vi "GenerateAlotOfSignals.vi"() -> (2 "DAQ":T1 {"data" format="%.2f"; "status" format="%08x"})   [LabVIEW 2014]
doc: "Generate some DAQ data (should later be the benchmark) to test the data historian."
uses:
  HISW/controls/typedef_PAQsample.ctl
  <vilib>/ptbypt/NI_PtbyPt.lvlib
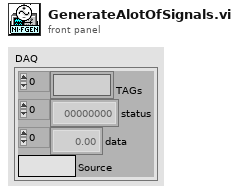
[diagram p1: front panel]
types:
  T1 = typedef "typedef_PAQsample.ctl" = cluster{"TAGs":string[], "status":u32[], "data":dbl[], "Source":string}
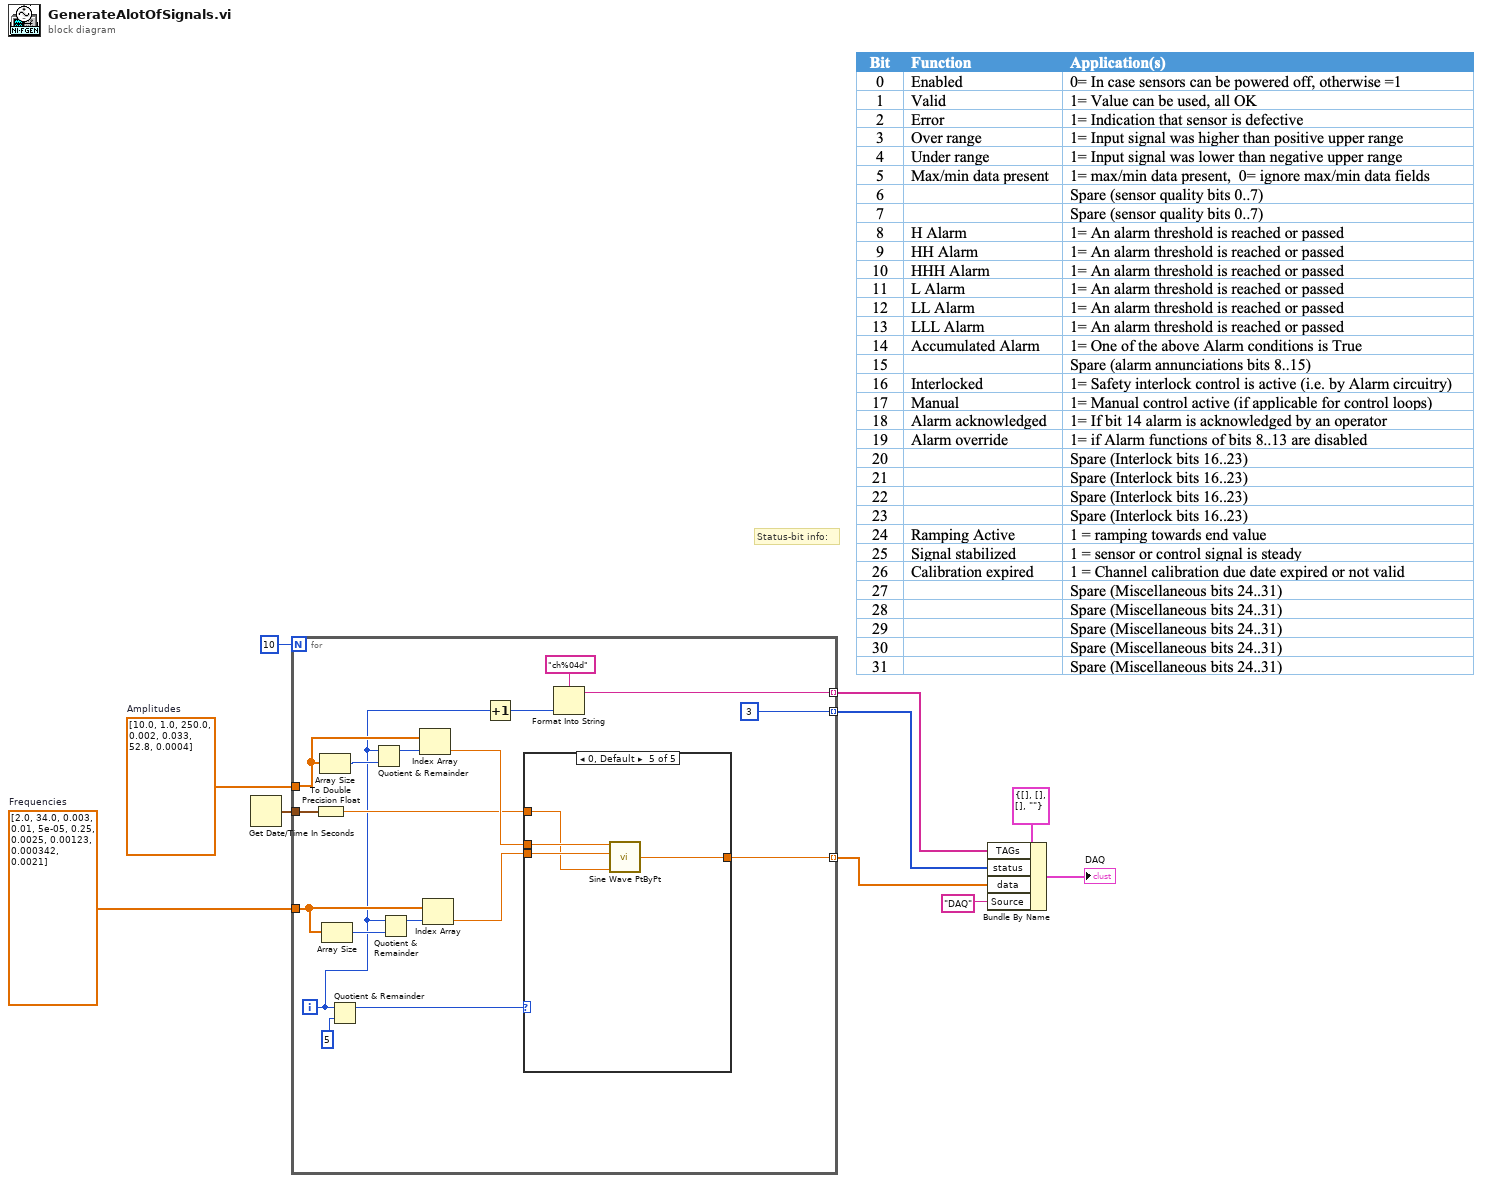
[diagram p0: block diagram]
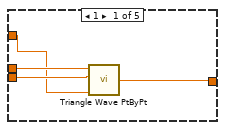
[diagram p2: hidden frame]
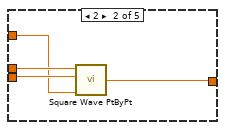
[diagram p3: hidden frame]
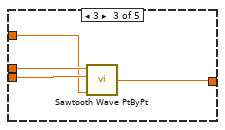
[diagram p4: hidden frame]
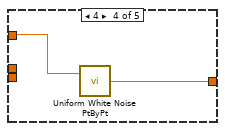
[diagram p5: hidden frame]
diagram:
  w9 = dbl[] [10.0, 1.0, 250.0, 0.002, 0.033, 52.8, 0.0004]  # Amplitudes
  w8 = dbl[] [2.0, 34.0, 0.003, 0.01, 5e-05, 0.25, 0.0025, 0.00123, 0.000342, 0.0021]  # Frequencies
  # "Status-bit info:"
  n1 = Get Date/Time In Seconds() -> (seconds since 1Jan1904=w7:timestamp)
  n2 = for {
    N: 10 -> [_]
    tunnel: w9 -> [w23]
    tunnel: w8 -> [w25]
    tunnel: w7 -> [w18]
    tunnel: [w16] -> w3 mode=indexing
    tunnel: [w12] -> w5 mode=indexing
    tunnel: [u32 3] -> w4 mode=indexing
    i -> [w15]
    n3 = To Double Precision Float(number=w18) -> (double precision float=w17:dbl)
    n4 = Array Size(array=w23) -> (size(s)=w26:i32)
    n5 = Array Size(array=w25) -> (size(s)=w27:i32)
    n6 = Quotient & Remainder(x=w15, y=5) -> (x-y*floor(x/y)=w21:i32)  [unwired: 1 out]
    n7 = Quotient & Remainder(x=w15, y=w26) -> (x-y*floor(x/y)=w22:i32)  [unwired: 1 out]
    n8 = Quotient & Remainder(x=w15, y=w27) -> (x-y*floor(x/y)=w24:i32)  [unwired: 1 out]
    n9 = Index Array(array=w23, index=w22) -> (element=w20:dbl)
    n10 = Index Array(array=w25, index=w24) -> (element=w19:dbl)
    n11 = Increment(x=w15) -> (x+1=w14:i32)
    n12 = case shown="0, Default" w21 {
      tunnel: w20 -> [w32 w36 w40 _ w46]
      tunnel: w19 -> [w31 w34 w39 _ w45]
      tunnel: w17 -> [w30 w33 w38 w42 w44]
      tunnel: [w29 w35 w37 w41 w43] -> w16
      frame 1 {
        n13 = call <vilib>:"Triangle Wave PtByPt.vi"("time"=w30, "frequency"=w31, "amplitude"=w32) -> ("triangle wave"=w29:dbl)  [unwired: 1 in]
      }
      frame 2 {
        n14 = call <vilib>:"Square Wave PtByPt.vi"("amplitude"=w36, "frequency"=w34, "time"=w33) -> ("square wave"=w35:dbl)  [unwired: 2 in]
      }
      frame 3 {
        n15 = call <vilib>:"Sawtooth Wave PtByPt.vi"("time"=w38, "frequency"=w39, "amplitude"=w40) -> ("sawtooth wave"=w37:dbl)  [unwired: 1 in]
      }
      frame 4 {
        n16 = call <vilib>:"Uniform White Noise PtByPt.vi"("amplitude"=w42) -> ("uniform white noise"=w41:dbl)  [unwired: 2 in]
      }
      frame 0, Default {
        n17 = call <vilib>:"Sine Wave PtByPt.vi"("time"=w44, "frequency"=w45, "amplitude"=w46) -> ("sine wave"=w43:dbl)  [unwired: 1 in]
      }
    }
    n18 = Format Into String(format string="ch%04d", w14) -> (resulting string=w12:string)  [unwired: 2 in, 1 out]
  }
  n19 = Bundle By Name(cluster=T1 {"TAGs"=[], "status"=[], "data"=[], "Source"=""} ("PAQsample"), "TAGs"=w5, "status"=w4, "data"=w3, "Source"="DAQ") -> (→"DAQ":T1)
